vi "Read dY_dX.vi"(8 "error in (no error)":errorcluster, 11 "IV_data in":refnum<class "IV_data.lvclass">) -> (0 "error out":errorcluster, 2 "dY/dX":dbl[](array[numeric]), 3 "IV_data out":refnum<class "IV_data.lvclass">)   [LabVIEW 2018, in "IV_data.lvclass"]
uses:
  IV_data.lvclass
  IV_data.lvclass/IV_data.ctl
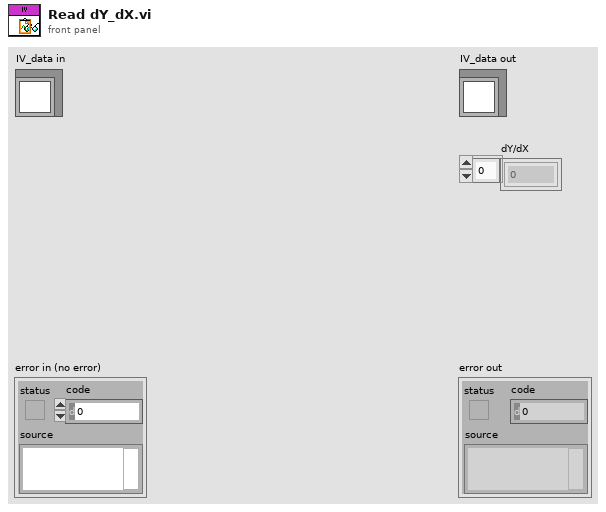
[diagram p1: front panel]
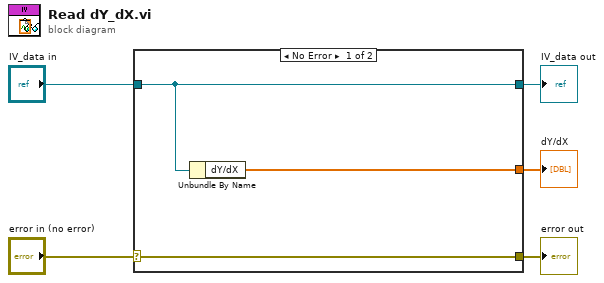
[diagram p0: block diagram]
diagram:
  n1 = case shown="No Error" "error in (no error)" {
    selector: "error in (no error)" -> [w8 w9]
    tunnel: [w8 w9] -> w4
    tunnel: [w7 w10] -> w2
    tunnel: "IV_data in" -> [w7 w10]
    tunnel: [w6 _] -> w1
    frame No Error {
      n2 = Unbundle By Name(w7) -> ("dY/dX"=w6:dbl[])
    }
    frame Error {
    }
  }
  "error out" <- w4
  "IV_data out" <- w2
  "dY/dX" <- w1
